vi "Write_rootURL.vi"(8 "error in":errorcluster, 10 "Root_URL":string, 11 "URL IN":T1) -> (0 "error out":errorcluster, 3 "URL OUT":T1)   [LabVIEW 2016]
uses:
  URL_Data.ctl
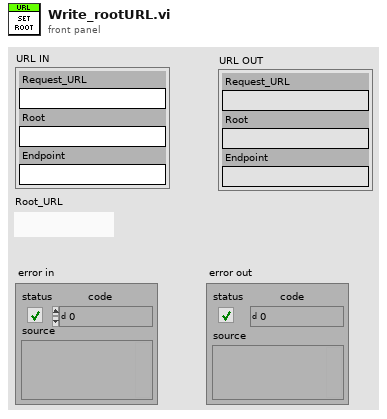
[diagram p1: front panel]
types:
  T1 = typedef "URL_Data.ctl" = cluster{"Root":string, "Endpoint":string, "Request_URL":string}
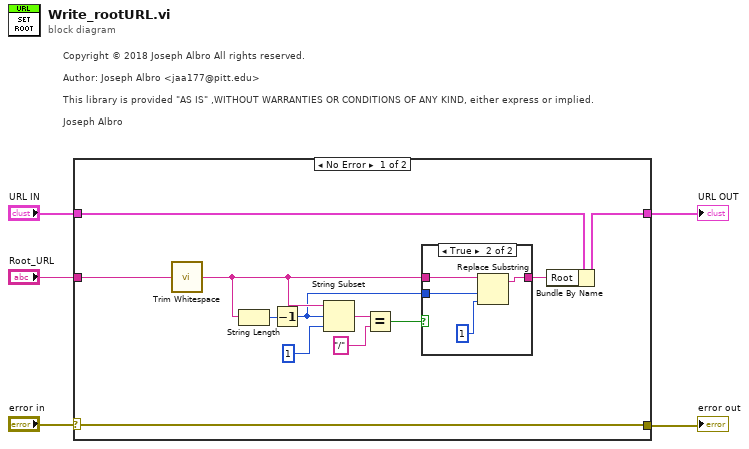
[diagram p0: block diagram]
diagram:
  # "Copyright © 2018 Joseph Albro All rights reserved.\n\nAuthor: Joseph Albro <jaa177@pitt.edu>\n\nThis library is provided \"AS IS\" ,WITHOUT WARRANTIES OR CONDITIONS OF ANY KIND, either express or implied.\n\nJoseph Albro"
  n1 = case shown="No Error" "error in" {
    selector: "error in" -> [w17 w24]
    tunnel: [w17 w24] -> w4
    tunnel: "URL IN" -> [w16 w23]
    tunnel: [w15 w23] -> w1
    tunnel: "Root_URL" -> [w13 _]
    frame No Error {
      n2 = call <vilib>:"Trim Whitespace.vi"("string"=w13) -> ("trimmed string"=w9:string)  [unwired: 1 in]
      n3 = String Length(string=w9) -> (length=w14:i32)
      n4 = Decrement(x=w14) -> (x-1=w7:i32)
      n5 = String Subset(string=w9, offset (0)=w7, length (rest)=1 ("length (rest)")) -> (substring=w12:string)
      n6 = Equal?(x=w12, y="/") -> (x = y?=w10:bool)
      n7 = case shown="True" w10 {
        tunnel: w9 -> [w18 w21]
        tunnel: w7 -> [_ w22]
        tunnel: [w18 w20] -> w8
        frame False {
        }
        frame True {
          n8 = Replace Substring(2:1 ("length (len. of substring)"), 3:w22, 5:w21) -> (1:w20:string)  [unwired: 1 in, 1 out]
        }
      }
      n9 = Bundle By Name(cluster=w16, "Root"=w8) -> (w15:T1)
    }
    frame Error {
    }
  }
  "error out" <- w4
  "URL OUT" <- w1
